vi "Setup Item Symbols.vi"(8 "error in (no error)":errorcluster, 11 "Selector in":refnum<class "Selector.lvclass">) -> (0 "error out":errorcluster, 3 "Selector out":refnum<class "Selector.lvclass">)   [LabVIEW 2019, in "Selector.lvclass"]
uses:
  Selector.lvclass
  <vilib>/picture/picture.llb/imagedata.ctl
  Selector.lvclass/Selector.ctl
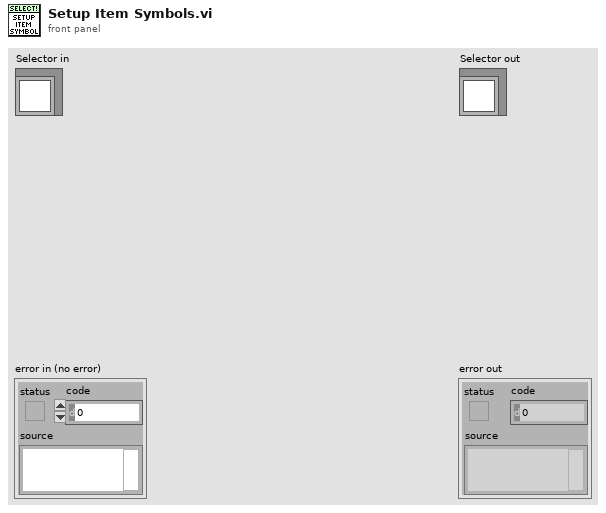
[diagram p1: front panel]
types:
  T1 = typedef "imagedata.ctl" = cluster{"image type":i32, "image depth":i32, "image":u8[], "mask":u8[], "colors":u32[], "Rectangle":cluster{"left":i16, "top":i16, "right":i16, "bottom":i16}}
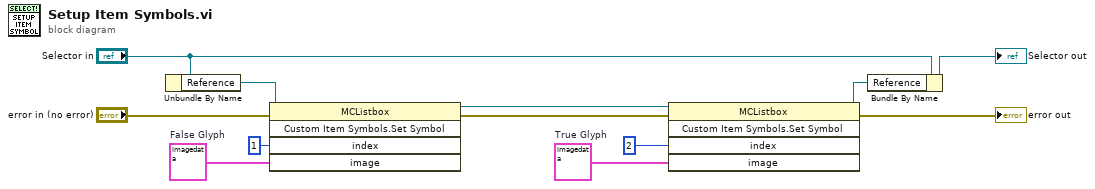
[diagram p0: block diagram]
diagram:
  w6 = T1 {"image type"=0, "image depth"=24, "image"=[255, 255, 255, 255, 255, 255, 255, 255, 255, 255, 255, 255, 255, 255, 255, 255, 255, 255, 255, 255, 255, 255, 255, 255, 255, 255, 255, 255, 255, 255, 255, 255, 255, 255, 255, 255, 255, 255, 255, 255, 255, 255, 255, 255, 255, 255, 255, 255, 255, 255, 255, 255, 255, 255, 255, 255, 255, 255, 255, 255, 255, 255, 255, 255, 255, 255, 255, 255, 255, 255, 255, 255, 255, 255, 255, 255, 255, 255, 255, 255, 255, 255, 255, 255, 255, 255, 255, 255, 255, 255, 255, 255, 255, 255, 255, 255, 255, 255, 255, 255, 255, 255, 255, 255, 255, 255, 255, 255, 181, 181, 181, 181, 181, 181, 181, 181, 181, 181, 181, 181, 181, 181, 181, 181, 181, 181, 181, 181, 181, 181, 181, 181, 255, 255, 255, 255, 255, 255, 255, 255, 255, 255, 255, 255, 255, 255, 255, 255, 255, 255, 255, 255, 255, 181, 181, 181, 100, 255, 0, 100, 255, 0, 100, 255, 0, 100, 255, 0, 100, 255, 0, 100, 255, 0, 100, 255, 0, 100, 255, 0, 181, 181, 181, 255, 255, 255, 255, 255, 255, 255, 255, 255, 255, 255, 255, 255, 255, 255, 181, 181, 181, 100, 255, 0, 100, 255, 0, 100, 255, 0, 100, 255, 0, 100, 255, 0, 100, 255, 0, 100, 255, 0, 100, 255, 0, 100, 255, 0, 100, 255, 0, 181, 181, 181, 255, 255, 255, 255, 255, 255, 255, 255, 255, 255, 255, 255, 181, 181, 181, 100, 255, 0, 100, 255, 0, 100, 255, 0, 100, 255, 0, 100, 255, 0, 100, 255, 0, 100, 255, 0, 100, 255, 0, 100, 255, 0, 100, 255, 0, 181, 181, 181, 255, 255, 255, 255, 255, 255, 255, 255, 255, 255, 255, 255, 181, 181, 181, 100, 255, 0, 100, 255, 0, 100, 255, 0, 100, 255, 0, 100, 255, 0, 100, 255, 0, 100, 255, 0, 100, 255, 0, 100, 255, 0, 100, 255, 0, 181, 181, 181, 255, 255, 255, 255, 255, 255, 255, 255, 255, 255, 255, 255, 181, 181, 181, 100, 255, 0, 100, 255, 0, 100, 255, 0, 100, 255, 0, 100, 255, 0, 100, 255, 0, 100, 255, 0, 100, 255, 0, 100, 255, 0, 100, 255, 0, 181, 181, 181, 255, 255, 255, 255, 255, 255, 255, 255, 255, 255, 255, 255, 181, 181, 181, 100, 255, 0, 100, 255, 0, 100, 255, 0, 100, 255, 0, 100, 255, 0, 100, 255, 0, 100, 255, 0, 100, 255, 0, 100, 255, 0, 100, 255, 0, 181, 181, 181, 255, 255, 255, 255, 255, 255, 255, 255, 255, 255, 255, 255, 181, 181, 181, 100, 255, 0, 100, 255, 0, 100, 255, 0, 100, 255, 0, 100, 255, 0, 100, 255, 0, 100, 255, 0, 100, 255, 0, 100, 255, 0, 100, 255, 0, 181, 181, 181, 255, 255, 255, 255, 255, 255, 255, 255, 255, 255, 255, 255, 181, 181, 181, 100, 255, 0, 100, 255, 0, 100, 255, 0, 100, 255, 0, 100, 255, 0, 100, 255, 0, 100, 255, 0, 100, 255, 0, 100, 255, 0, 100, 255, 0, 181, 181, 181, 255, 255, 255, 255, 255, 255, 255, 255, 255, 255, 255, 255, 181, 181, 181, 100, 255, 0, 100, 255, 0, 100, 255, 0, 100, 255, 0, 100, 255, 0, 100, 255, 0, 100, 255, 0, 100, 255, 0, 100, 255, 0, 100, 255, 0, 181, 181, 181, 255, 255, 255, 255, 255, 255, 255, 255, 255, 255, 255, 255, 255, 255, 255, 181, 181, 181, 100, 255, 0, 100, 255, 0, 100, 255, 0, 100, 255, 0, 100, 255, 0, 100, 255, 0, 100, 255, 0, 100, 255, 0, 181, 181, 181, 255, 255, 255, 255, 255, 255, 255, 255, 255, 255, 255, 255, 255, 255, 255, 255, 255, 255, 255, 255, 255, 181, 181, 181, 181, 181, 181, 181, 181, 181, 181, 181, 181, 181, 181, 181, 181, 181, 181, 181, 181, 181, 181, 181, 181, 255, 255, 255, 255, 255, 255, 255, 255, 255, 255, 255, 255, 255, 255, 255, 255, 255, 255, 255, 255, 255, 255, 255, 255, 255, 255, 255, 255, 255, 255, 255, 255, 255, 255, 255, 255, 255, 255, 255, 255, 255, 255, 255, 255, 255, 255, 255, 255, 255, 255, 255, 255, 255, 255, 255, 255, 255, 255, 255, 255, 255, 255, 255, 255, 255, 255, 255, 255, 255, 255, 255, 255, 255, 255, 255, 255, 255, 255, 255, 255, 255, 255, 255, 255, 255, 255, 255, 255, 255, 255, 255, 255, 255, 255, 255, 255, 255, 255, 255, 255, 255, 255, 255, 255, 255, 255, 255, 255], "mask"=[], "colors"=[], "Rectangle"={"left"=0, "top"=0, "right"=16, "bottom"=16}}  # True Glyph
  w9 = T1 {"image type"=0, "image depth"=24, "image"=[255, 255, 255, 255, 255, 255, 255, 255, 255, 255, 255, 255, 255, 255, 255, 255, 255, 255, 255, 255, 255, 255, 255, 255, 255, 255, 255, 255, 255, 255, 255, 255, 255, 255, 255, 255, 255, 255, 255, 255, 255, 255, 255, 255, 255, 255, 255, 255, 255, 255, 255, 255, 255, 255, 255, 255, 255, 255, 255, 255, 255, 255, 255, 255, 255, 255, 255, 255, 255, 255, 255, 255, 255, 255, 255, 255, 255, 255, 255, 255, 255, 255, 255, 255, 255, 255, 255, 255, 255, 255, 255, 255, 255, 255, 255, 255, 255, 255, 255, 255, 255, 255, 255, 255, 255, 255, 255, 255, 181, 181, 181, 181, 181, 181, 181, 181, 181, 181, 181, 181, 181, 181, 181, 181, 181, 181, 181, 181, 181, 181, 181, 181, 255, 255, 255, 255, 255, 255, 255, 255, 255, 255, 255, 255, 255, 255, 255, 255, 255, 255, 255, 255, 255, 181, 181, 181, 240, 240, 240, 240, 240, 240, 240, 240, 240, 240, 240, 240, 240, 240, 240, 240, 240, 240, 240, 240, 240, 240, 240, 240, 181, 181, 181, 255, 255, 255, 255, 255, 255, 255, 255, 255, 255, 255, 255, 255, 255, 255, 181, 181, 181, 240, 240, 240, 240, 240, 240, 240, 240, 240, 240, 240, 240, 240, 240, 240, 240, 240, 240, 240, 240, 240, 240, 240, 240, 240, 240, 240, 240, 240, 240, 181, 181, 181, 255, 255, 255, 255, 255, 255, 255, 255, 255, 255, 255, 255, 181, 181, 181, 240, 240, 240, 240, 240, 240, 240, 240, 240, 240, 240, 240, 240, 240, 240, 240, 240, 240, 240, 240, 240, 240, 240, 240, 240, 240, 240, 240, 240, 240, 181, 181, 181, 255, 255, 255, 255, 255, 255, 255, 255, 255, 255, 255, 255, 181, 181, 181, 240, 240, 240, 240, 240, 240, 240, 240, 240, 240, 240, 240, 240, 240, 240, 240, 240, 240, 240, 240, 240, 240, 240, 240, 240, 240, 240, 240, 240, 240, 181, 181, 181, 255, 255, 255, 255, 255, 255, 255, 255, 255, 255, 255, 255, 181, 181, 181, 240, 240, 240, 240, 240, 240, 240, 240, 240, 240, 240, 240, 240, 240, 240, 240, 240, 240, 240, 240, 240, 240, 240, 240, 240, 240, 240, 240, 240, 240, 181, 181, 181, 255, 255, 255, 255, 255, 255, 255, 255, 255, 255, 255, 255, 181, 181, 181, 240, 240, 240, 240, 240, 240, 240, 240, 240, 240, 240, 240, 240, 240, 240, 240, 240, 240, 240, 240, 240, 240, 240, 240, 240, 240, 240, 240, 240, 240, 181, 181, 181, 255, 255, 255, 255, 255, 255, 255, 255, 255, 255, 255, 255, 181, 181, 181, 240, 240, 240, 240, 240, 240, 240, 240, 240, 240, 240, 240, 240, 240, 240, 240, 240, 240, 240, 240, 240, 240, 240, 240, 240, 240, 240, 240, 240, 240, 181, 181, 181, 255, 255, 255, 255, 255, 255, 255, 255, 255, 255, 255, 255, 181, 181, 181, 240, 240, 240, 240, 240, 240, 240, 240, 240, 240, 240, 240, 240, 240, 240, 240, 240, 240, 240, 240, 240, 240, 240, 240, 240, 240, 240, 240, 240, 240, 181, 181, 181, 255, 255, 255, 255, 255, 255, 255, 255, 255, 255, 255, 255, 181, 181, 181, 240, 240, 240, 240, 240, 240, 240, 240, 240, 240, 240, 240, 240, 240, 240, 240, 240, 240, 240, 240, 240, 240, 240, 240, 240, 240, 240, 240, 240, 240, 181, 181, 181, 255, 255, 255, 255, 255, 255, 255, 255, 255, 255, 255, 255, 255, 255, 255, 181, 181, 181, 240, 240, 240, 240, 240, 240, 240, 240, 240, 240, 240, 240, 240, 240, 240, 240, 240, 240, 240, 240, 240, 240, 240, 240, 181, 181, 181, 255, 255, 255, 255, 255, 255, 255, 255, 255, 255, 255, 255, 255, 255, 255, 255, 255, 255, 255, 255, 255, 181, 181, 181, 181, 181, 181, 181, 181, 181, 181, 181, 181, 181, 181, 181, 181, 181, 181, 181, 181, 181, 181, 181, 181, 255, 255, 255, 255, 255, 255, 255, 255, 255, 255, 255, 255, 255, 255, 255, 255, 255, 255, 255, 255, 255, 255, 255, 255, 255, 255, 255, 255, 255, 255, 255, 255, 255, 255, 255, 255, 255, 255, 255, 255, 255, 255, 255, 255, 255, 255, 255, 255, 255, 255, 255, 255, 255, 255, 255, 255, 255, 255, 255, 255, 255, 255, 255, 255, 255, 255, 255, 255, 255, 255, 255, 255, 255, 255, 255, 255, 255, 255, 255, 255, 255, 255, 255, 255, 255, 255, 255, 255, 255, 255, 255, 255, 255, 255, 255, 255, 255, 255, 255, 255, 255, 255, 255, 255, 255, 255, 255, 255], "mask"=[], "colors"=[], "Rectangle"={"left"=0, "top"=0, "right"=16, "bottom"=16}}  # False Glyph
  n1 = Unbundle By Name("Selector in") -> ("Reference"=w2:refnum<vi>)
  n2 = invoke class="MCListbox" method="Custom Item Symbols.Set Symbol"(reference=w2, error in="error in (no error)", "index"=1 ("Index"), "image"=w9) -> (reference out=w8:refnum<vi>, error out=w5:errorcluster)  [unwired: 1 in, 3 out]
  n3 = invoke class="MCListbox" method="Custom Item Symbols.Set Symbol"(reference=w8, error in=w5, "index"=2 ("Index"), "image"=w6) -> (reference out=w1:refnum<vi>, error out=→"error out":errorcluster)  [unwired: 1 in, 3 out]
  n4 = Bundle By Name(cluster="Selector in", "Reference"=w1) -> (→"Selector out":refnum<class "Selector.lvclass">)
